vi "SetParam.vi"(8 "error in (no error)":errorcluster caption="entrée d'erreur (pas d'erreur)", 10 "power_transform":T1={"method"="yeo-johnson", "standardize"=TRUE, "copy"=TRUE}, 11 "power_transform.lvclass":refnum<class "power_transform.lvclass">) -> (0 "error out":errorcluster caption="sortie d'erreur", 3 "power_transform.lvclass":refnum<class "power_transform.lvclass">)   [LabVIEW 2020, in "power_transform.lvclass"]
doc: "Set Parameters"
uses:
  power_transform.lvclass
  power_transform.lvclass/power_transform.ctl
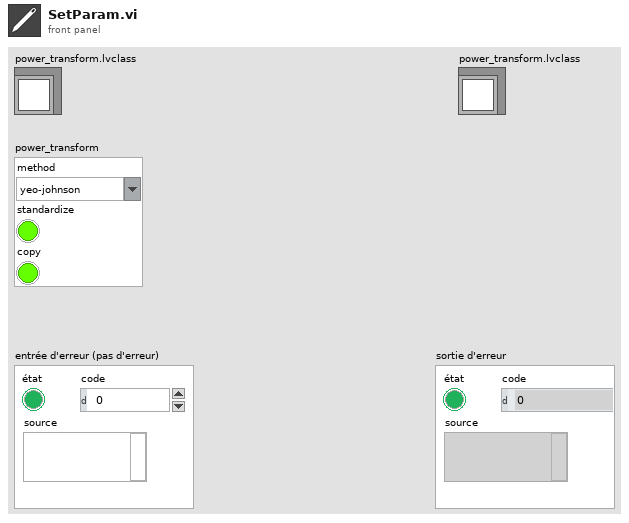
[diagram p1: front panel]
types:
  T1 = cluster{"method":string, "standardize":bool, "copy":bool}
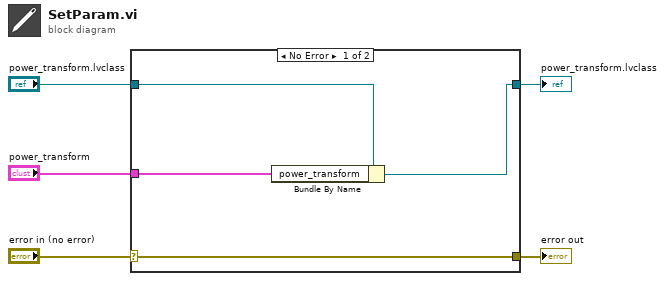
[diagram p0: block diagram]
diagram:
  n1 = case shown="No Error" "error in (no error)" {
    selector: "error in (no error)" -> [w9 w10]
    tunnel: [w9 w10] -> w4
    tunnel: [w7 w11] -> w2
    tunnel: "power_transform.lvclass" -> [w8 w11]
    tunnel: "power_transform" -> [w6 _]
    frame No Error {
      n2 = Bundle By Name(cluster=w8, "power_transform"=w6) -> (w7:refnum<class "power_transform.lvclass">)
    }
    frame Error {
    }
  }
  "error out" <- w4
  "power_transform.lvclass" <- w2
